vi "PID.vi"(0 "PID":cluster{"Kp":dbl, "1/Ti":dbl, "Td":dbl}, 1 "Current Velocity":dbl, 2 "Ref. Velocity":dbl, 3 "tk-1":cluster{"Ik-1":dbl, "erk-1":dbl}) -> (5 "Uk":dbl, 8 "tk":cluster{" Ik":dbl, "erk":dbl})   [LabVIEW 2016]
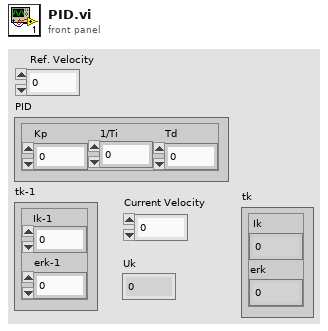
[diagram p1: front panel]
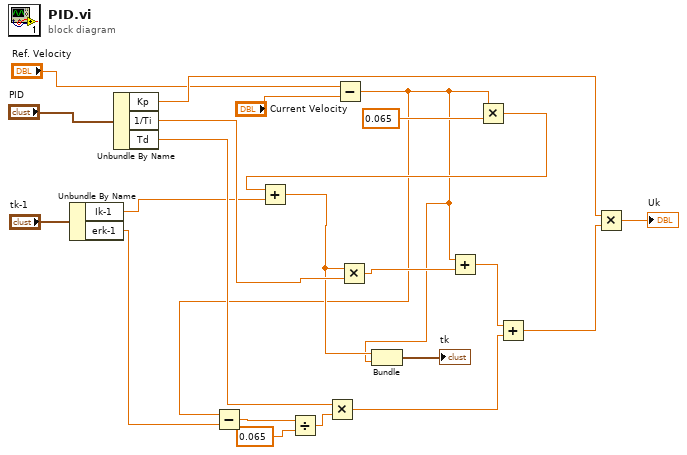
[diagram p0: block diagram]
diagram:
  n1 = Unbundle By Name("tk-1") -> ("Ik-1"=w6:dbl, "erk-1"=w5:dbl)
  n2 = Unbundle By Name("PID") -> ("Kp"=w10:dbl, "1/Ti"=w9:dbl, "Td"=w11:dbl)
  n3 = Subtract(x="Ref. Velocity", y="Current Velocity") -> (x-y=w2:dbl)
  n4 = Subtract(x=w2, y=w5) -> (x-y=w20:dbl)
  n5 = Divide(x=w20, y=0.065) -> (x/y=w21:dbl)
  n6 = Multiply(x=w11, y=w21) -> (x*y=w19:dbl)
  n7 = Multiply(x=w2, y=0.065) -> (x*y=w13:dbl)
  n8 = Add(x=w13, y=w6) -> (x+y=w3:dbl)
  n9 = Multiply(x=w3, y=w9) -> (x*y=w12:dbl)
  n10 = Bundle(w3, w2) -> (→"tk":cluster{dbl, dbl})  [unwired: 1 in]
  n11 = Add(x=w2, y=w12) -> (x+y=w18:dbl)
  n12 = Add(x=w18, y=w19) -> (x+y=w16:dbl)
  n13 = Multiply(x=w10, y=w16) -> (x*y=→"Uk":dbl)
